vi "mtg - check which to update.vi"(9 "graph selection":T1(ring)=enum."5 hr", 10 "update times":i32[](array[numeric])=[1, 5, 30, 60, 120], 11 "iteration index (s)":i32) -> (3 "update list (10...)":i32[](array[numeric]))   [LabVIEW 2025]
panel:
  # "graph on display\n\n1 s\n\n5 s\n\n30 s\n\n60 s\n\n120 s"
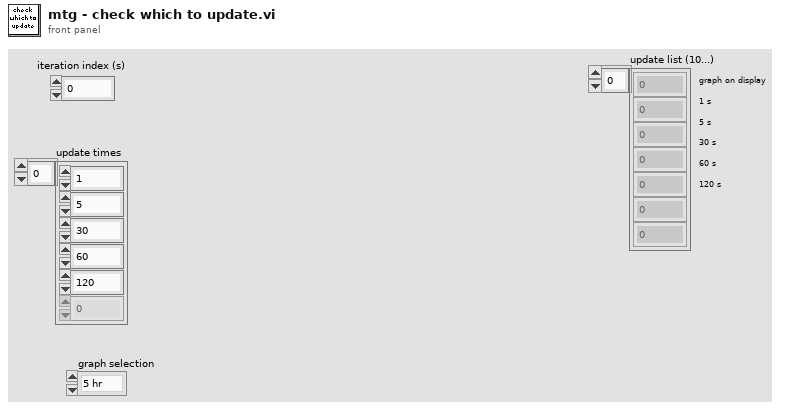
[diagram p1: front panel]
types:
  T1 = enum16{"1 hr", "5 hr", "30 hr", "60 hr", "120 hr", "1 hr (from file)"}
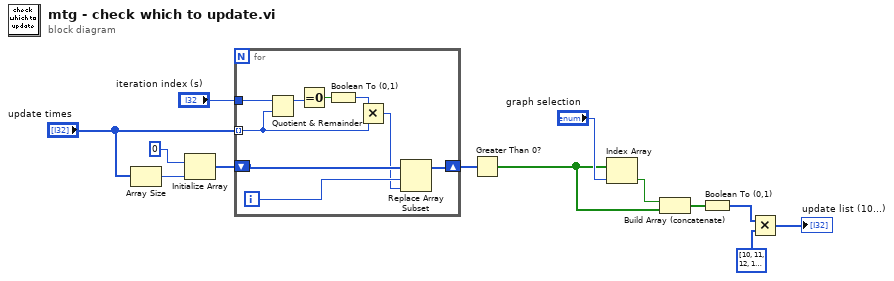
[diagram p0: block diagram]
diagram:
  n1 = Array Size(array="update times") -> (size(s)=w11:i32)
  n2 = Initialize Array(0, w11) -> (w9:i32[])
  n3 = for {
    tunnel: "iteration index (s)" -> [w19]
    tunnel: "update times" -> [w18] mode=indexing
    shift-right: [w14] -> w8
    shift-left: w9 -> [w17]
    i -> [w16]
    n4 = Quotient & Remainder(x=w19, y=w18) -> (x-y*floor(x/y)=w22:i32)  [unwired: 1 out]
    n5 = Equal To 0?(x=w22) -> (x = 0?=w20:bool)
    n6 = Boolean To (0,1)(Boolean=w20) -> (0, 1=w21:i16)
    n7 = Multiply(x=w21, y=w18) -> (x*y=w15:i32)
    n8 = Replace Array Subset(array=w17, new element=w15, index=w16) -> (w14:i32[])
  }
  n9 = Greater Than 0?(x=w8) -> (x > 0?=w5:bool[])
  n10 = Index Array(array=w5, index="graph selection") -> (element=w6:bool)
  n11 = Build Array (concatenate)(w6, w5) -> (w4:bool[])
  n12 = Boolean To (0,1)(Boolean=w4) -> (0, 1=w3:i16[])
  n13 = Multiply(x=w3, y=i16[] [10, 11, 12, 13, 14, 15, 16, 17, 18, 19, 20] ("x")) -> (x*y=→"update list (10...)":i16[])
